vi "Add LRC.vi"(8 "error in (no error)":errorcluster, 11 "String in":string) -> (0 "error out":errorcluster, 3 "String":string)   [LabVIEW 2020, in "Protections.lvlib" / "LRC - HRZ Series.lvclass"]
uses:
  LRC - HRZ Series.lvclass
  LRC - HRZ Series.lvclass/LRC - HRZ Series.ctl
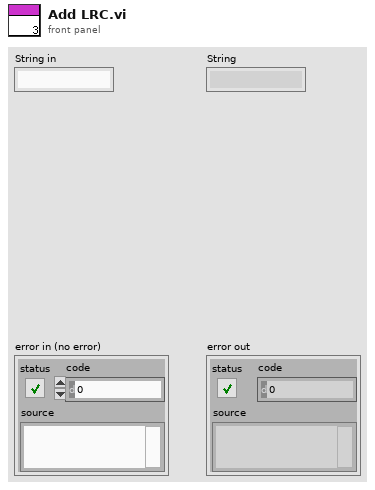
[diagram p1: front panel]
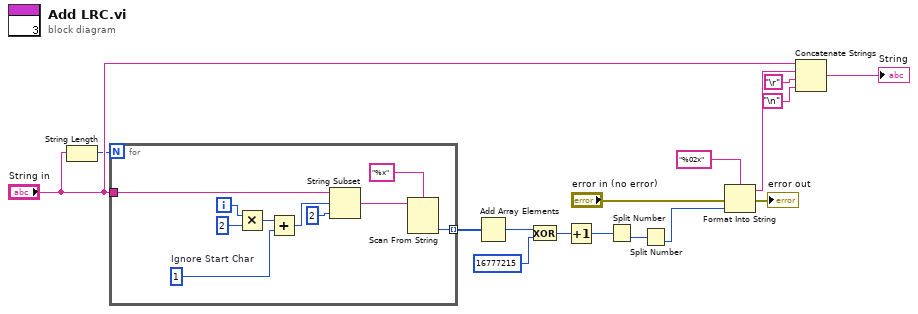
[diagram p0: block diagram]
diagram:
  n1 = String Length(string="String in") -> (length=w1:i32)
  n2 = for {
    N: w1 -> [_]
    tunnel: "String in" -> [w26]
    tunnel: [w19] -> w3 mode=indexing
    i -> [w25]
    w17 = 1  # Ignore Start Char
    n3 = Multiply(x=w25, y=2) -> (x*y=w24:i32)
    n4 = Add(x=w24, y=w17) -> (x+y=w18:i32)
    n5 = String Subset(string=w26, offset (0)=w18, length (rest)=2 ("length (rest)")) -> (substring=w21:string)
    n6 = Scan From String(format string="%x", input string=w21) -> (output 1=w19:u32)  [unwired: 3 in, 3 out]
  }
  n7 = Add Array Elements(numeric array=w3) -> (sum=w4:u32)
  n8 = Exclusive Or(1:u32 16777215 ("y"), 2:w4) -> (0:w6:u32)
  n9 = Increment(x=w6) -> (x+1=w7:u32)
  n10 = Split Number(x=w7) -> (lo(x)=w8:u16)  [unwired: 1 out]
  n11 = Split Number(x=w8) -> (lo(x)=w12:u8)  [unwired: 1 out]
  n12 = Format Into String(format string="%02x", error in="error in (no error)", w12) -> (resulting string=w14:string, error out=→"error out":errorcluster)  [unwired: 1 in]
  n13 = Concatenate Strings("String in", w14, "\r", "\n") -> (→"String":string)
